vi "Close Workspace Control Refs.vi"(11 "State Variables in":T1) -> ()   [LabVIEW 2015, in "Diagnostics Addon Shared.lvlib"]
uses:
  Diagnostics Addon Shared.lvlib
  Types/Workspace.State.ctl
  Types/UI.Refs.ctl
  Types/Command.ctl
  <vilib>/NI Veristand/Display Template Support/Display Template Support.llb/enum_Display Template Handler Minimal To Workspace.ctl
  Types/Workspace.SavedState.ctl
  NationalInstruments.VeriStand.SystemStorage
  <vilib>/NI Veristand/Execution/Workspace/WorkspaceAPI.ctl
  NationalInstruments.VeriStand.ClientAPI
  <vilib>/NI Veristand/Display Template Support/Display Template Support.llb/enum_Display Template Handler Minimal To Widget Msg.ctl
  <vilib>/NI Veristand/Execution/Workspace/SystemStateRegEventRef.ctl
  <vilib>/NI Veristand/Execution/Workspace/Target State Info.ctl
  <vilib>/NI Veristand/Execution/Workspace/Target State.ctl
  <vilib>/NI Veristand/Execution/Workspace/SystemStateEventRef.ctl
  Types/Protocol.ctl
  <vilib>/NI Veristand/Execution/Workspace/NI_VS Workspace ExecutionAPI.lvlib
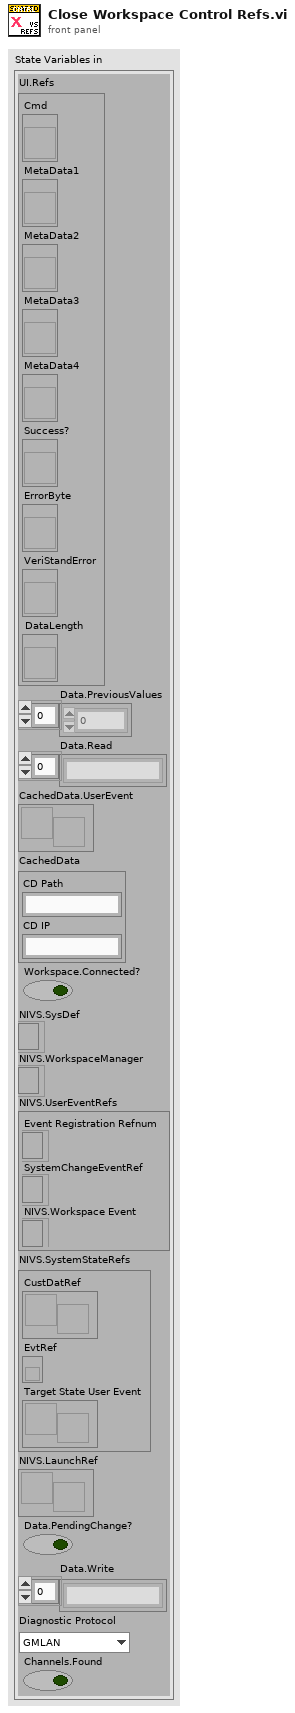
[diagram p1: front panel]
types:
  T1 = typedef "Diagnostics Addon Shared.lvlib/Workspace.State.ctl" = cluster{"UI.Refs":T2, "Data.PreviousValues":dbl[], "Data.Read":string[], "CachedData.UserEvent":refnum<user-event>, "CachedData":T3, "Workspace.Connected?":bool, "NIVS.SysDef":refnum<k24>, "NIVS.WorkspaceManager":T4, "NIVS.UserEventRefs":cluster{"Event Registration Refnum":refnum<event-registration>, "SystemChangeEventRef":T5, "NIVS.Workspace Event":refnum<event-registration>}, "NIVS.SystemStateRefs":T6, "NIVS.LaunchRef":refnum<user-event>, "Data.PendingChange?":bool, "Data.Write":string[], "Diagnostic Protocol":T7, "Channels.Found":bool}
  T2 = typedef "Diagnostics Addon Shared.lvlib/UI.Refs.ctl" = cluster{"Cmd":refnum<vi>, "MetaData1":refnum<vi>, "MetaData2":refnum<vi>, "MetaData3":refnum<vi>, "MetaData4":refnum<vi>, "Success?":refnum<vi>, "ErrorByte":refnum<vi>, "VeriStandError":refnum<vi>, "DataLength":refnum<vi>}
  T3 = typedef "Diagnostics Addon Shared.lvlib/Workspace.SavedState.ctl" = cluster{"CD Path":string, "CD IP":string}
  T4 = typedef "NI_VS Workspace ExecutionAPI.lvlib/WorkspaceAPI.ctl" = refnum<k24>
  T5 = typedef "NI_VS Workspace ExecutionAPI.lvlib/SystemStateRegEventRef.ctl" = refnum<event-registration>
  T6 = typedef "NI_VS Workspace ExecutionAPI.lvlib/SystemStateEventRef.ctl" = cluster{"CustDatRef":refnum<user-event>, "EvtRef":refnum<k27>, "Target State User Event":refnum<user-event>}
  T7 = typedef "Diagnostics Addon Shared.lvlib/Protocol.ctl" = enum16{"GMLAN", "KWP-2000", "UDS"}
  T8 = cluster{"Event Registration Refnum":refnum<event-registration>, "SystemChangeEventRef":T5, "NIVS.Workspace Event":refnum<event-registration>}
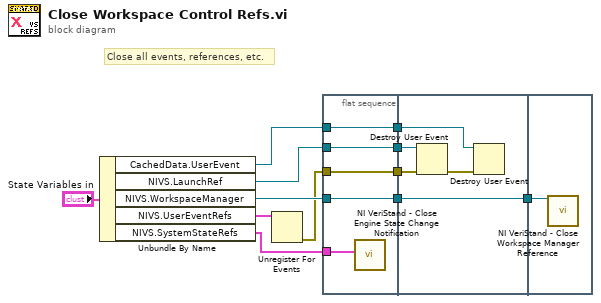
[diagram p0: block diagram]
diagram:
  # "Close all events, references, etc."
  n1 = Unbundle By Name("State Variables in") -> ("CachedData.UserEvent"=w7:refnum<user-event>, "NIVS.LaunchRef"=w6:refnum<user-event>, "NIVS.WorkspaceManager"=w4:T4, "NIVS.UserEventRefs"=w3:T8, "NIVS.SystemStateRefs"=w5:T6)
  n2 = Unregister For Events(event registration refnum=w3) -> (error out=w1:errorcluster)  [unwired: 1 in]
  n3 = flat-sequence {
    tunnel: w4 -> [w14]
    tunnel: w5 -> [w13]
    tunnel: w7 -> [w15]
    tunnel: w6 -> [w16]
    tunnel: w1 -> [w17]
    tunnel: [w17] -> w12
    tunnel: [w16] -> w11
    tunnel: [w15] -> w10
    tunnel: [w14] -> w9
    tunnel: w12 -> [w21]
    tunnel: w11 -> [w22]
    tunnel: w10 -> [w19]
    tunnel: w9 -> [w18]
    tunnel: [w18] -> w8
    tunnel: w8 -> [w23]
    frame #0 {
      n4 = call <vilib>:"NI VeriStand - Close Engine State Change Notification.vi"("SystemStateRefs"=w13) -> ()  [unwired: 10 in, 1 out]
    }
    frame #1 {
      n5 = Destroy User Event(user event=w22, error in=w21) -> (error out=w20:errorcluster)
      n6 = Destroy User Event(user event=w19, error in=w20) -> ()  [unwired: 1 out]
    }
    frame #2 {
      n7 = call <vilib>:"NI VeriStand - Close Workspace Manager Reference.vi"("WorkspaceManager"=w23) -> ()  [unwired: 10 in, 1 out]
    }
  }
